vi "HV_power_supply_set_voltage.vi"(7 "error in":errorcluster, 8 "Desired output voltage in V (HV power supply)":dbl, 10 "Channel of HV power supply":refnum<k21>) -> (0 "error out":errorcluster)   [LabVIEW 2009]
uses:
  <vilib>/ULx/Write.llb/ULx Write (Analog 1D DBL 1Chan 1Samp).vi
  <vilib>/ULx/Create Channel.llb/ULx Create Channel (AO-Voltage-Basic).vi
panel:
  in  "Max. voltage in V (HV power supply)":dbl=2000.0
  in  "Max. voltage in V (Redlab box)":dbl=4.0
  # "Input"
  # "Constants"
  # "Caution! Changing these constants might cause \na dangerous change in the high voltage output!"
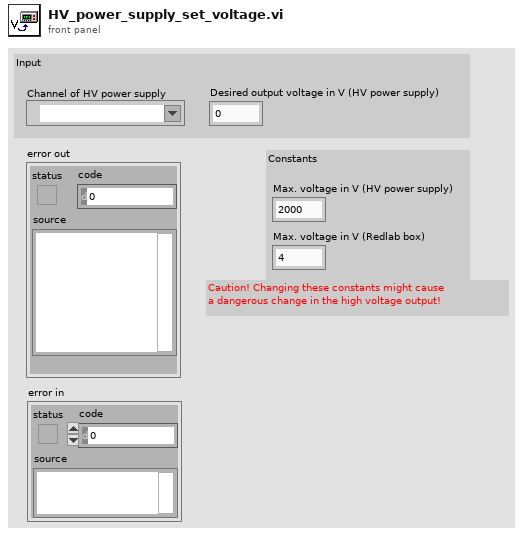
[diagram p1: front panel]
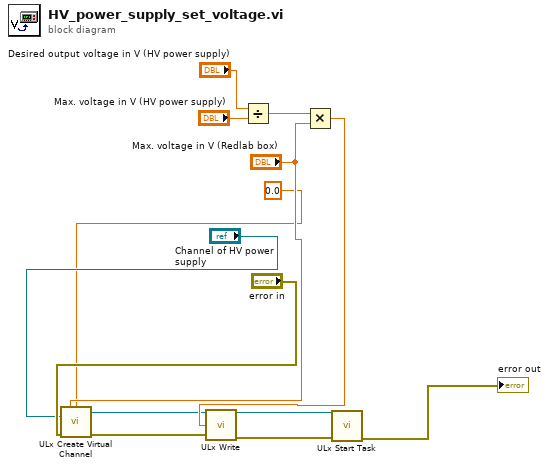
[diagram p0: block diagram]
diagram:
  n1 = call-poly <vilib>:"ULx Create Virtual Channel.vi"("maximum value"="Max. voltage in V (Redlab box)", "minimum value"=0.0, "physical channels"="Channel of HV power supply", "error in"="error in") -> ("task out"=w3:refnum<k24>, "error out"=w10:errorcluster)  [unwired: 10 in]
  n2 = Divide(x="Desired output voltage in V (HV power supply)", y="Max. voltage in V (HV power supply)") -> (x/y=w13:dbl)
  n3 = Multiply(x=w13, y="Max. voltage in V (Redlab box)") -> (x*y=w4:dbl)
  n4 = call-poly <vilib>:"ULx Write.vi"("task in"=w3, "data"=w4, "error in"=w10) -> ("task out"=w2:refnum<k24>, "error out"=w9:errorcluster)  [unwired: 10 in, 1 out]
  n5 = call <vilib>:"ULx Start Task.vi"("task in"=w2, "error in"=w9) -> ("error out"=→"error out":errorcluster)  [unwired: 12 in, 1 out]
